vi "Path_String_Splitter.vi"(3 "File Path":path) -> (0 "Session Name":string, 1 "Experiment Name":string)   [LabVIEW 2023]
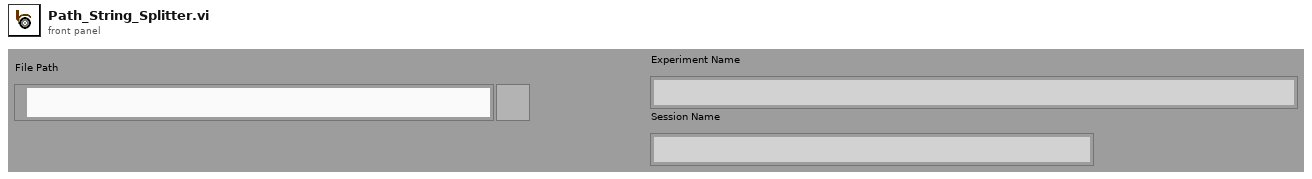
[diagram p1: front panel]
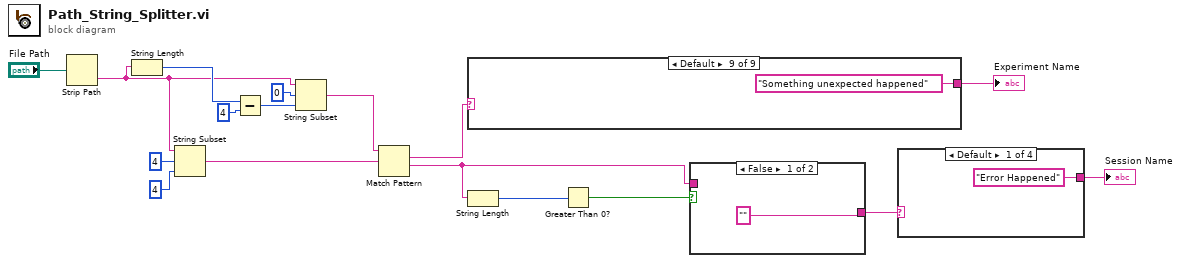
[diagram p0: block diagram]
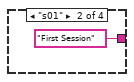
[diagram p2: hidden frame]
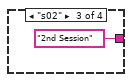
[diagram p3: hidden frame]
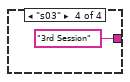
[diagram p4: hidden frame]
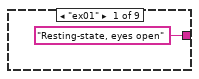
[diagram p5: hidden frame]
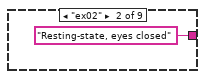
[diagram p6: hidden frame]
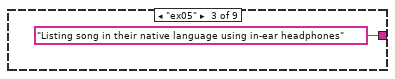
[diagram p7: hidden frame]
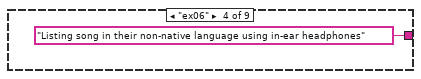
[diagram p8: hidden frame]
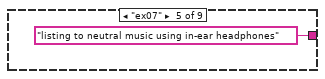
[diagram p9: hidden frame]
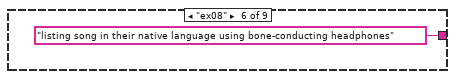
[diagram p10: hidden frame]
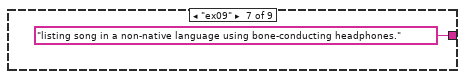
[diagram p11: hidden frame]
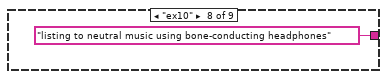
[diagram p12: hidden frame]
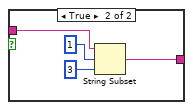
[diagram p13: hidden frame]
diagram:
  n1 = Strip Path(path="File Path") -> (name=w8:string)  [unwired: 1 out]
  n2 = String Length(string=w8) -> (length=w15:i32)
  n3 = String Subset(string=w8, offset (0)=4, length (rest)=4 ("length (rest)")) -> (substring=w5:string)
  n4 = Subtract(x=w15, y=4) -> (x-y=w17:i32)
  n5 = String Subset(string=w8, offset (0)=0, length (rest)=w17) -> (substring=w14:string)
  n6 = Match Pattern(string=w14, regular expression=w5) -> (match substring=w2:string, after substring=w11:string)  [unwired: 1 in, 2 out]
  n7 = case shown="Default" w2 {
    tunnel: ["Resting-state, eyes open" "Resting-state, eyes closed" "Listing song in their native language using in-ear headphones" "Listing song in their non-native language using in-ear headphones" "listing to neutral music using in-ear headphones" "listing song in their native language using bone-conducting headphones" "listing song in a non-native language using bone-conducting headphones." "listing to neutral music using bone-conducting headphones" "Something unexpected happened"] -> w4
    frame "ex01" {
    }
    frame "ex02" {
    }
    frame "ex05" {
    }
    frame "ex06" {
    }
    frame "ex07" {
    }
    frame "ex08" {
    }
    frame "ex09" {
    }
    frame "ex10" {
    }
    frame Default {
    }
  }
  "Experiment Name" <- w4
  n8 = String Length(string=w11) -> (length=w10:i32)
  n9 = Greater Than 0?(x=w10) -> (x > 0?=w9:bool)
  n10 = case shown="False" w9 {
    tunnel: w11 -> [_ w29]
    tunnel: ["" w28] -> w1
    frame False {
    }
    frame True {
      n11 = String Subset(string=w29, offset (0)=1, length (rest)=3 ("length (rest)")) -> (substring=w28:string)
    }
  }
  n12 = case shown="Default" w1 {
    tunnel: ["Error Happened" "First Session" "2nd Session" "3rd Session"] -> w3
    frame Default {
    }
    frame "s01" {
    }
    frame "s02" {
    }
    frame "s03" {
    }
  }
  "Session Name" <- w3
